vi "EXA shm accept Command Set Value LV.vi"(8 "error in (no error)":errorcluster, 11 "command_SetValue_Ctl":cluster{"size":i32, "data":string}) -> (0 "error out":errorcluster, 2 "function return":i32, 3 "command_SetValue_Ctl out":cluster{"size":i32, "data":string})   [LabVIEW 2016, in "SALLV_EXA.lvlib"]
doc: "int EXA_shm_acceptCommand_SetValueLV(EXA_command_SetValueLV *command_SetValue_Ctl );"
uses:
  SALLV_EXA.lvlib
  SALLV_EXA.so
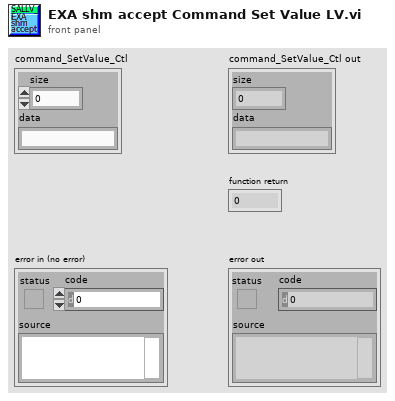
[diagram p1: front panel]
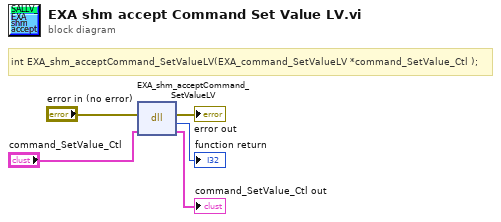
[diagram p0: block diagram]
diagram:
  # "int EXA_shm_acceptCommand_SetValueLV(EXA_command_SetValueLV *command_SetValue_Ctl );"
  n1 = dll-call lib="home/plotz/SALLV_EXA/SALLV_EXA.*" fn="EXA_shm_acceptCommand_SetValueLV"(error in="error in (no error)", "command_SetValue_Ctl"="command_SetValue_Ctl") -> (error out=→"error out":errorcluster, →"function return":i32, "command_SetValue_Ctl"=→"command_SetValue_Ctl out":cluster{"size":i32, "data":string})  [unwired: 2 in, 1 out]
